vi "Reset Slit.vi"(8 "error in (no error)":errorcluster, 10 "Slit":T1(ring), 11 "VISA resource name":refnum<visa-resource-name>) -> (0 "error out":errorcluster, 3 "VISA resource name out":refnum<visa-resource-name>)   [LabVIEW 2009, in "Digikrom DK24x.lvlib"]
doc: "This command returns one or all slits to the home position.\n\n0: All Slits\n1: Entrance Slit\n2: Exit Slit\n3: Middle Slit (DK242 only)"
uses:
  Digikrom DK24x.lvlib
  Private/Command.ctl
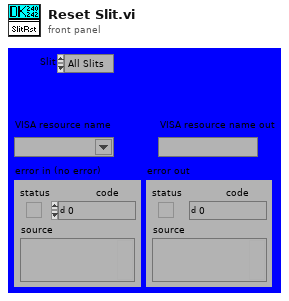
[diagram p1: front panel]
types:
  T1 = enum8{"All Slits", "Entrance Slit", "Exit Slit", "Middle Slit (DK242 Only)"}
  T2 = typedef "Digikrom DK24x.lvlib/Command.ctl" = u8
  T3 = enum8{"All Slits", "Entrance Slit", "Exit Slit", "Middle Slit (DK242 Only)"}[]
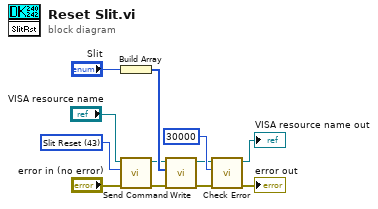
[diagram p0: block diagram]
diagram:
  w1 = T2 43 items=["Cancel"=24, "Clear"=25, "CSR"=28, "Echo"=27, "Filter"=15, "Gcal"=18, "Goto"=16, "Grtid?"=19, "Grtsel"=26, "NOVRAM Read"=56, "NOVRAM Write"=59, "Reset"=255, "Scan"=12, "Scan Up"=9, "Scan Down"=3, "Serial?"=33, "Slew Up"=8, "Slew Down"=2, "Slit Reset"=43, "Slit?"=30, "Sltadj"=14, "Speed"=13, "Sspeed?"=21, "Step Down"=1, "Step Up"=7, "S1adj"=31, "S2adj"=32, "S3adj"=34, "S1cal"=22, "S2cal"=23, "S3cal"=35, "Test"=17, "Type"=57, "Wave?"=29, "Zero"=52] ("Command")
  n1 = Build Array("Slit") -> (w12:T3)
  n2 = call "Send Command.vi"("error in (no error)"="error in (no error)", "Command"=w1, "VISA resource name"="VISA resource name") -> ("error out"=w7:errorcluster, "VISA resource name out"=w8:refnum<visa-resource-name>)  [unwired: 7 out]
  n3 = call "Write.vi"("error in (no error)"=w7, "Byte Array"=w12, "VISA resource name"=w8) -> ("error out"=w4:errorcluster, "VISA resource name out"=w5:refnum<visa-resource-name>)  [unwired: 7 out]
  n4 = call "Check Error.vi"("error in"=w4, "timeout"=u32 30000, "VISA resource name in"=w5) -> ("error out"=→"error out":errorcluster, "VISA resource name out"=→"VISA resource name out":refnum<visa-resource-name>)  [unwired: 7 out]
